vi "SBG_Ellipse_starting_debug (SubVI) (1).vi"(10 "boolean from check":bool, 11 "result string in":string) -> (3 "result string out":string)   [LabVIEW 2017]
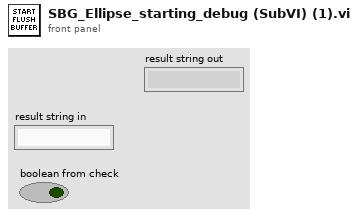
[diagram p1: front panel]
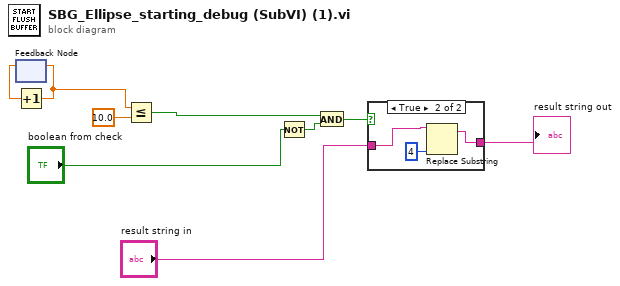
[diagram p0: block diagram]
diagram:
  n1 = feedback #1() -> (w2:dbl)  [unwired: 1 in]
  n2 = Increment(x=w2) -> (x+1=w1:dbl)
  n3 = feedback-in #1(w1) -> ()
  n4 = Less Or Equal?(x=w1, y=10.0) -> (x <= y?=w3:bool)
  n5 = Not(x="boolean from check") -> (.not. x?=w7:bool)
  n6 = And(x=w3, y=w7) -> (x .and. y?=w6:bool)
  n7 = case shown="True" w6 {
    tunnel: "result string in" -> [w10 w11]
    tunnel: [w10 w12] -> w9
    frame False {
    }
    frame True {
      n8 = Replace Substring(2:4 ("length (len. of substring)"), 5:w11) -> (1:w12:string)  [unwired: 2 in, 1 out]
    }
  }
  "result string out" <- w9
